vi "Process ASCII Data.vi"(11 "data":u8[](array[numeric])) -> (3 "pdu":u8[](array[numeric]))   [LabVIEW 2012, in "ASCII Data Unit.lvclass"]
uses:
  ASCII Data Unit.lvclass
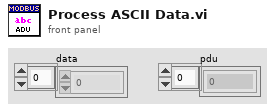
[diagram p1: front panel]
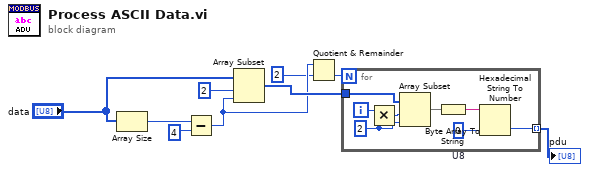
[diagram p0: block diagram]
diagram:
  n1 = Array Size(array="data") -> (size(s)=w2:i32)
  n2 = Subtract(x=w2, y=4) -> (x-y=w7:i32)
  n3 = Array Subset(array="data", index=2, length=w7) -> (w8:u8[])
  n4 = Quotient & Remainder(x=w7, y=2) -> (floor(x/y)=w5:i32)  [unwired: 1 out]
  n5 = for {
    N: w5 -> [_]
    tunnel: [w12] -> w9 mode=indexing
    tunnel: w8 -> [w10]
    i -> [w17]
    w13 = u8 0  # U8
    w16 = 2 ("length")
    n6 = Multiply(x=w17, y=w16) -> (x*y=w15:i32)
    n7 = Array Subset(array=w10, index=w15, length=w16) -> (w11:u8[])
    n8 = Byte Array To String(unsigned byte array=w11) -> (string=w14:string)
    n9 = Hexadecimal String To Number(string=w14, default (0uL)=w13) -> (number=w12:u8)  [unwired: 2 out]
  }
  "pdu" <- w9
